vi "Single Random Bump.vi"(5 "Bump Parameters":T1={"Distance (deg)"=2.0, "Travel time (ms)"=500.0} {"Travel time (ms)" min=0.1 max=10000.0; "Distance (deg)" min=0.1}) -> ()   [LabVIEW 2010]
panel:
  out "concatenated string 2":string
  out "concatenated string":string
  out "Feedrate out":dbl
  out "degrees out":dbl
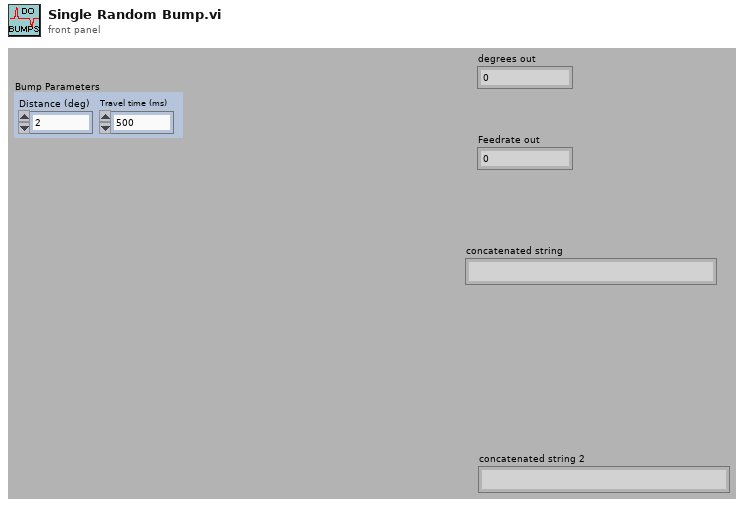
[diagram p1: front panel]
types:
  T1 = cluster{"Distance (deg)":dbl, "Travel time (ms)":dbl}
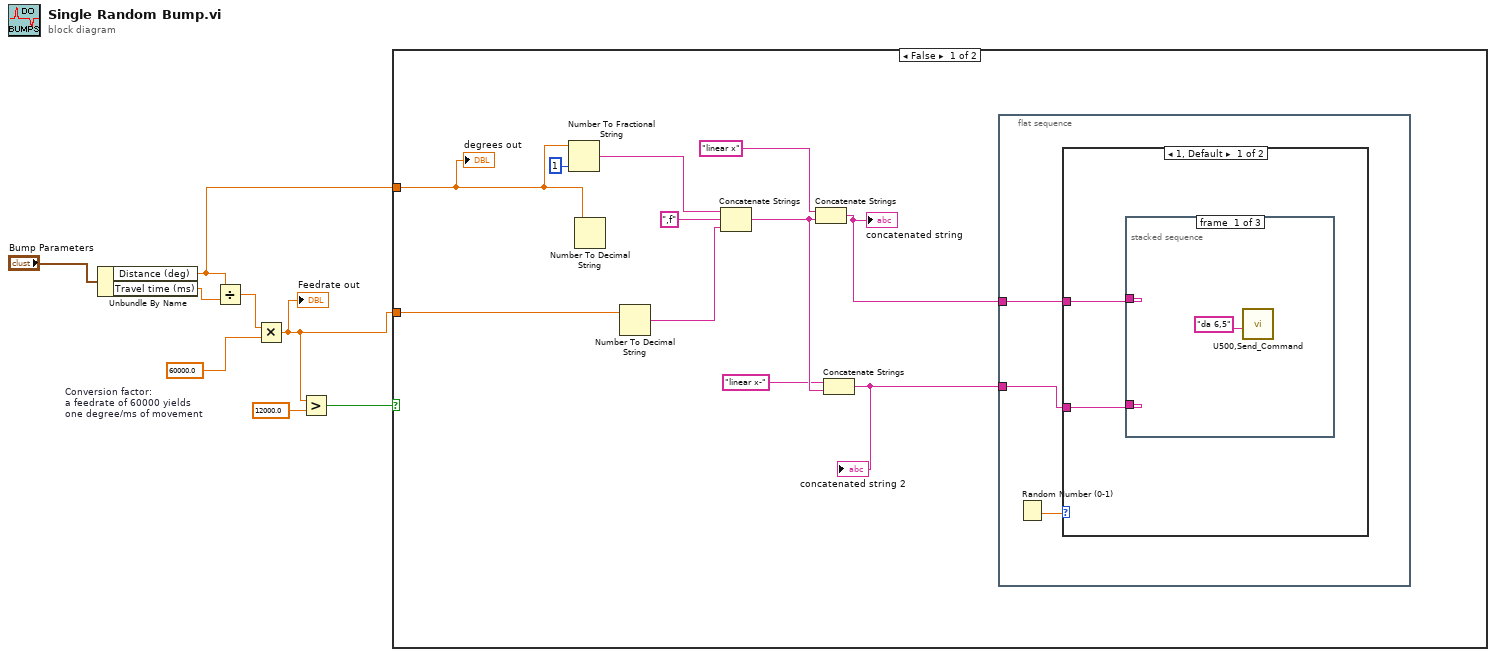
[diagram p0: block diagram]
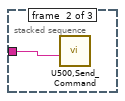
[diagram p2: hidden frame]
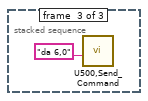
[diagram p3: hidden frame]
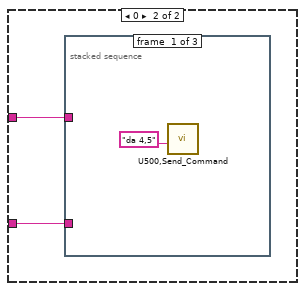
[diagram p4: hidden frame]
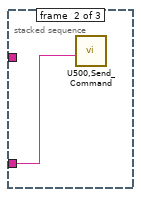
[diagram p5: hidden frame]
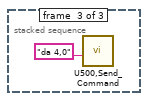
[diagram p6: hidden frame]
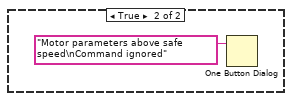
[diagram p7: hidden frame]
diagram:
  w5 = 60000.0  # Conversion factor: a feedrate of 60000 yields one degree/ms of movement
  n1 = Unbundle By Name("Bump Parameters") -> ("Distance (deg)"=w4:dbl, "Travel time (ms)"=w7:dbl)
  n2 = Divide(x=w4, y=w7) -> (x/y=w6:dbl)
  n3 = Multiply(x=w6, y=w5) -> (x*y=w3:dbl)
  "Feedrate out" <- w3
  n4 = Greater?(x=w3, y=12000.0) -> (0:w1:bool)
  n5 = case shown="False" w1 {
    tunnel: w4 -> [w12 _]
    tunnel: w3 -> [w9 _]
    frame False {
      n6 = Number To Fractional String(number=w12, precision (6)=i16 1) -> (F-format string=w11:string)  [unwired: 2 in]
      n7 = Number To Decimal String(number=w12) -> ()  [unwired: 1 in, 1 out]
      n8 = Number To Decimal String(number=w9) -> (decimal integer string=w18:string)  [unwired: 1 in]
      n9 = Concatenate Strings(w11, ",f" ("F-format string"), w18) -> (w16:string)
      n10 = Concatenate Strings("linear x" ("string"), w16) -> (w14:string)
      "concatenated string" <- w14
      n11 = Concatenate Strings("linear x-" ("string"), w16) -> (w13:string)
      "concatenated string 2" <- w13
      n12 = flat-sequence {
        tunnel: w14 -> [w22]
        tunnel: w13 -> [w21]
        frame #0 {
          n13 = Random Number (0-1)() -> (number: 0 to 1=w20:dbl)
          n14 = case shown="1, Default" w20 {
            tunnel: w22 -> [w24 w29]
            tunnel: w21 -> [w23 w28]
            frame 1, Default {
              n15 = stacked-sequence {
                tunnel: w24 -> [_ w26 _]
                tunnel: w23 -> [_ _ _]
                frame #0 {
                  n16 = call "U500,Send_Command.vi"("Command String"="da 6,5") -> ()  [unwired: 9 in, 2 out]
                }
                frame #1 {
                  n17 = call "U500,Send_Command.vi"("Command String"=w26) -> ()  [unwired: 9 in, 2 out]
                }
                frame #2 {
                  n18 = call "U500,Send_Command.vi"("Command String"="da 6,0") -> ()  [unwired: 9 in, 2 out]
                }
              }
            }
            frame 0 {
              n19 = stacked-sequence {
                tunnel: w29 -> [_ _ _]
                tunnel: w28 -> [_ w31 _]
                frame #0 {
                  n20 = call "U500,Send_Command.vi"("Command String"="da 4,5") -> ()  [unwired: 9 in, 2 out]
                }
                frame #1 {
                  n21 = call "U500,Send_Command.vi"("Command String"=w31) -> ()  [unwired: 9 in, 2 out]
                }
                frame #2 {
                  n22 = call "U500,Send_Command.vi"("Command String"="da 4,0") -> ()  [unwired: 9 in, 2 out]
                }
              }
            }
          }
        }
      }
      "degrees out" <- w12
    }
    frame True {
      n23 = One Button Dialog(message="Motor parameters above safe speed\nCommand ignored") -> ()  [unwired: 1 in, 1 out]
    }
  }
